vi "MeasAction.vi"(8 "error in (no error)":errorcluster caption="entrée d'erreur (pas d'erreur)", 9 "CurvePointIndex":i32, 10 "AllPointIndex":i32, 11 "InstrClassIn":refnum<class "AttoAMC.lvclass"> caption="DNL_LabVIEW Object in") -> (0 "error out":errorcluster caption="sortie d'erreur", 2 "MeasDatOut":dbl[](array[numeric]), 3 "InstrClassOut":refnum<class "AttoAMC.lvclass"> caption="DNL_LabVIEW Object out")   [LabVIEW 2019, in "AttoAMC.lvclass"]
uses:
  AttoAMC.lvclass
  AttoAMC.lvclass/AttoAMC.ctl
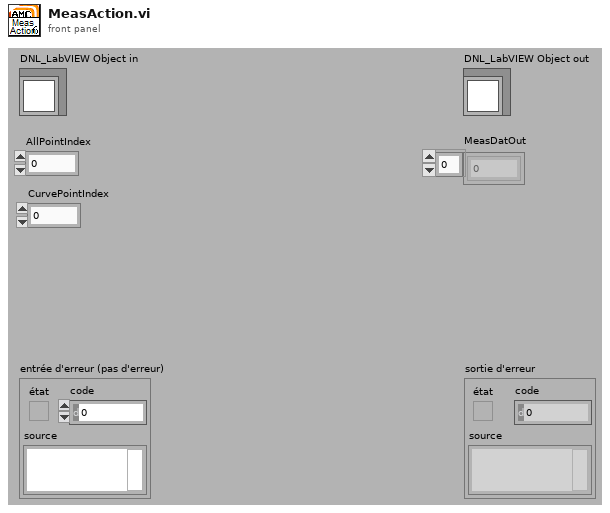
[diagram p1: front panel]
types:
  T1 = typedef "AttoAMC.lvclass/AttoAMC_Func.ctl" = enum16{"Position (um)"}
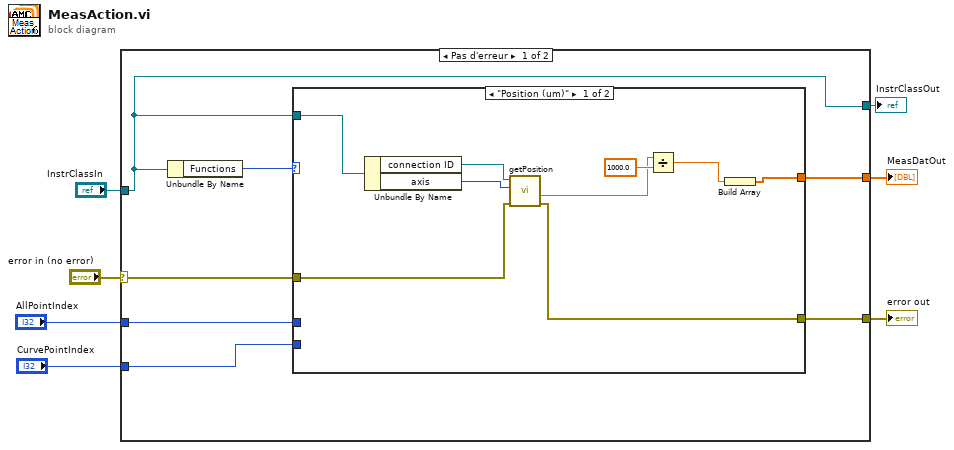
[diagram p0: block diagram]
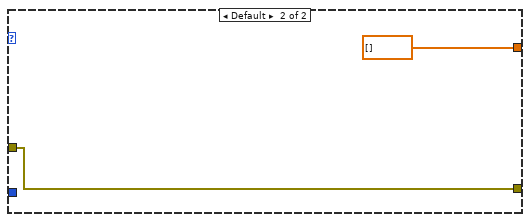
[diagram p2: hidden frame]
diagram:
  n1 = case shown="Pas d'erreur" "error in (no error)" {
    selector: "error in (no error)" -> [w10 w26]
    tunnel: "InstrClassIn" -> [w8 w27]
    tunnel: [w8 w27] -> w5
    tunnel: "AllPointIndex" -> [w14 _]
    tunnel: [w13 w26] -> w3
    tunnel: [w12 _] -> w2
    tunnel: "CurvePointIndex" -> [w9 _]
    frame No Error {
      n2 = Unbundle By Name(w8) -> ("Functions"=w11:T1)
      n3 = case shown="\"Position (um)\"" w11 {
        tunnel: w14 -> [_ _]
        tunnel: [w15 w25] -> w13
        tunnel: [w20 dbl[] [] ("Outputs")] -> w12
        tunnel: w10 -> [w16 w25]
        tunnel: w9 -> [_ _]
        tunnel: w8 -> [w23 _]
        frame "Position (um)" {
          n4 = Unbundle By Name(w23) -> ("connection ID"=w22:refnum<k5>, "axis"=w21:u8)
          n5 = call <userlib>:"getPosition.vi"("error in"=w16, "axis in"=w21, "connection ID"=w22) -> ("error out"=w15:errorcluster, "position out"=w17:dbl)  [unwired: 5 in, 2 out]
          n6 = Divide(x=w17, y=1000.0) -> (x/y=w19:dbl)
          n7 = Build Array(w19) -> (w20:dbl[])
        }
        frame Default {
        }
      }
    }
    frame Error {
    }
  }
  "error out" <- w3
  "InstrClassOut" <- w5
  "MeasDatOut" <- w2
